vi "ISX3_Cmd_SetSetupAddFrequency.vi"(1 "Use LogScale":bool, 5 "Start Frequency [Hz]":sgl=0.01 min=0.01 max=1e+07, 7 "Stop Frequency [Hz]":sgl=0.01 min=0.01 max=1e+07, 9 "Frequency Count":sgl=1.0 min=1 max=2048 step=1, 12 "Precision":sgl min=0, 13 "Amplitude [V]":sgl=0.01 min=0.001 max=1) -> (10 "set Setup Init Cmd":u8[](array[numeric]) format="%x")   [LabVIEW 2012, in "Sciospec ISX3 Impedance Analyzer.lvlib"]
uses:
  Sciospec ISX3 Impedance Analyzer.lvlib
panel:
  # "This VI generates the command to initate a new frequency block in the system."
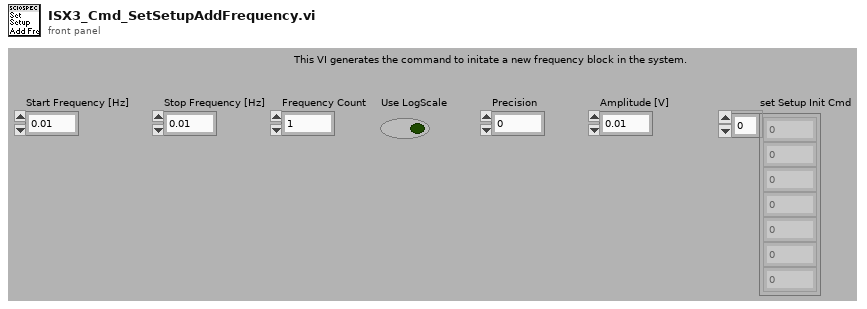
[diagram p1: front panel]
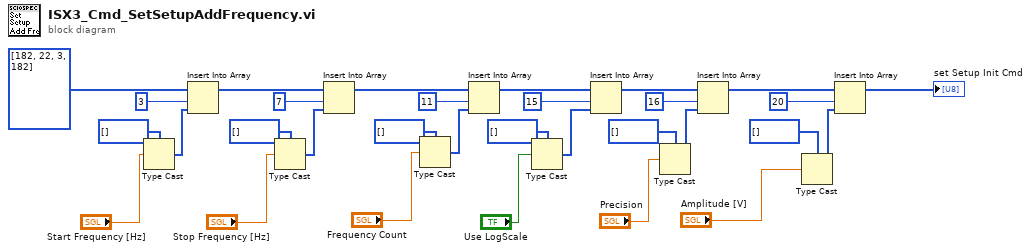
[diagram p0: block diagram]
diagram:
  n1 = Type Cast(type=u8[] [], x="Start Frequency [Hz]") -> (*(type *) &x=w28:u8[])
  n2 = Insert Into Array(array=u8[] [182, 22, 3, 182], index=3, new element=w28) -> (w26:u8[])
  n3 = Type Cast(type=u8[] [], x="Stop Frequency [Hz]") -> (*(type *) &x=w21:u8[])
  n4 = Insert Into Array(array=w26, index=7, new element=w21) -> (w4:u8[])
  n5 = Type Cast(type=u8[] [], x="Frequency Count") -> (*(type *) &x=w6:u8[])
  n6 = Insert Into Array(array=w4, index=11, new element=w6) -> (w3:u8[])
  n7 = Type Cast(type=u8[] [], x="Use LogScale") -> (*(type *) &x=w18:u8[])
  n8 = Insert Into Array(array=w3, index=15, new element=w18) -> (w25:u8[])
  n9 = Type Cast(type=u8[] [], x="Precision") -> (*(type *) &x=w14:u8[])
  n10 = Insert Into Array(array=w25, index=16, new element=w14) -> (w24:u8[])
  n11 = Type Cast(type=u8[] [], x="Amplitude [V]") -> (*(type *) &x=w10:u8[])
  n12 = Insert Into Array(array=w24, index=20, new element=w10) -> (→"set Setup Init Cmd":u8[])
